vi "Meas_Sweep.vi"(0 "SPU":refnum<k24>, 1 "Flag_215":bool, 2 "MPM":refnum<k24>[](array[refnum]), 3 "Data_struct":refnum<k24>[](array[refnum]), 4 "TSL":refnum<k24>, 5 "错误输入（无错误）":errorcluster, 7 "ILSTS":refnum<k24>, 8 "Flag_213":bool, 11 "Meas_monitor_struct":refnum<k24>[](array[refnum]), 12 "Meas_rang":i32[](array[numeric])) -> (19 "错误输出":errorcluster)   [LabVIEW 2017]
uses:
  D:/test/ILSTS/LV_IL_Sample/DLL/InstrumentDLL.dll
  DLL/InstrumentDLL.dll
  D:/test/ILSTS/LV_IL_Sample/DLL/STSProcess.dll
  DLL/STSProcess.dll
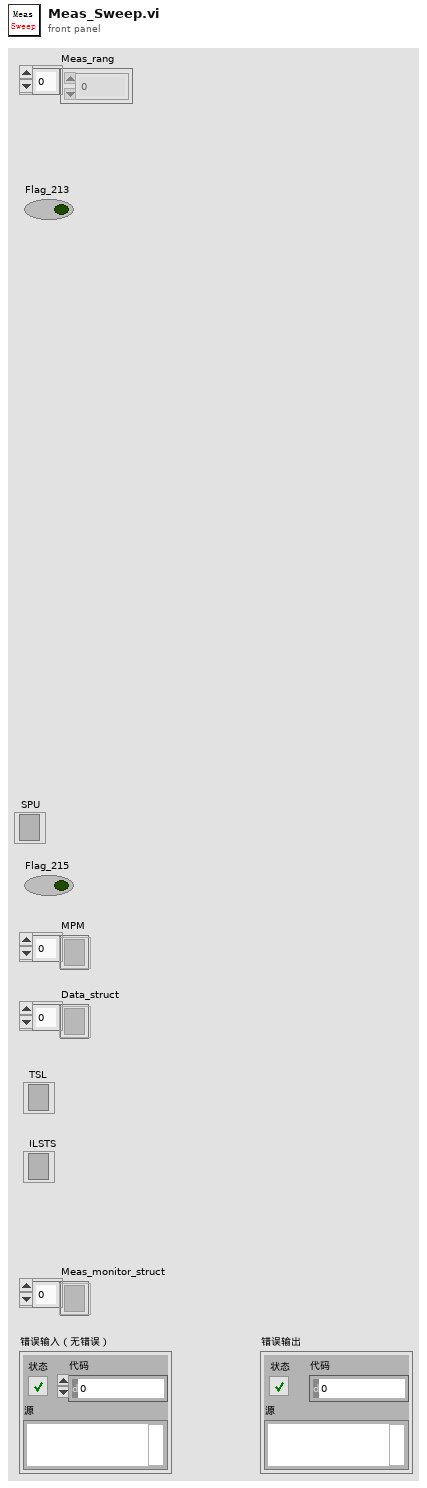
[diagram p1: front panel]
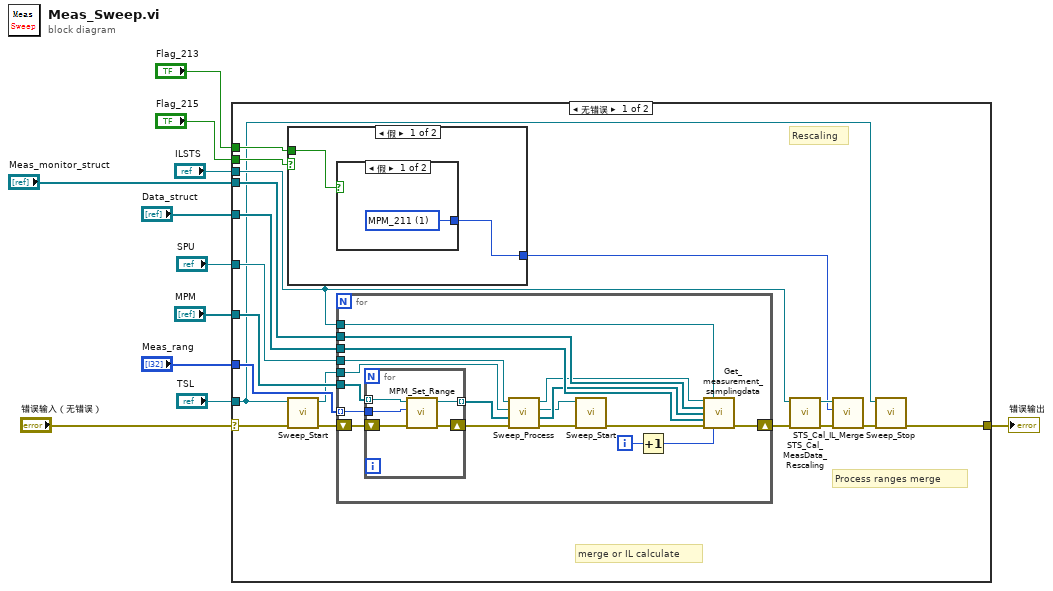
[diagram p0: block diagram]
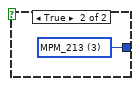
[diagram p2: hidden frame]
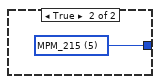
[diagram p3: hidden frame]
diagram:
  n1 = case shown="无错误" "错误输入（无错误）" {
    selector: "错误输入（无错误）" -> [w19 w58]
    tunnel: [w29 w58] -> w11
    tunnel: "Flag_213" -> [w28 _]
    tunnel: "Flag_215" -> [w27 _]
    tunnel: "MPM" -> [w26 _]
    tunnel: "Data_struct" -> [w25 _]
    tunnel: "Meas_monitor_struct" -> [w24 _]
    tunnel: "SPU" -> [w23 _]
    tunnel: "ILSTS" -> [w22 _]
    tunnel: "Meas_rang" -> [w21 _]
    tunnel: "TSL" -> [w20 _]
    frame No Error {
      # "Rescaling"
      # "Process ranges merge"
      # "merge or IL calculate"
      n2 = case shown="假" w27 {
        tunnel: [w31 w34] -> w13
        tunnel: w28 -> [w30 _]
        frame False {
          n3 = case shown="假" w30 {
            tunnel: [w32 w33] -> w31
            frame False {
              w32 = 1 items=["MPM_10"=0, "MPM_211"=1, "MPM_212"=2, "MPM_213"=3, "MPM_215"=5] ("type")
            }
            frame True {
              w33 = 3 items=["MPM_10"=0, "MPM_211"=1, "MPM_212"=2, "MPM_213"=3, "MPM_215"=5] ("type")
            }
          }
        }
        frame True {
          w34 = 5 items=["MPM_10"=0, "MPM_211"=1, "MPM_212"=2, "MPM_213"=3, "MPM_215"=5] ("type")
        }
      }
      n4 = call "Sweep_Start.vi"("error in (no error)"=w19, ".NET Reference in"=w20) -> ("error out"=w18:errorcluster, "Reference out"=w17:refnum<k24>)  [unwired: 8 in]
      n5 = for {
        tunnel: w21 -> [w51] mode=indexing
        tunnel: w26 -> [w43]
        tunnel: w17 -> [w48]
        tunnel: w23 -> [w44]
        tunnel: w22 -> [w47]
        tunnel: w24 -> [w46]
        tunnel: w25 -> [w45]
        shift-right: [w42] -> w12
        shift-left: w18 -> [w52]
        i -> [w41]
        n6 = for {
          tunnel: w43 -> [w57] mode=indexing
          tunnel: w51 -> [w54]
          shift-right: [w55] -> w50
          shift-left: w52 -> [w56]
          tunnel: [w53] -> w40 mode=indexing
          n7 = call "MPM_Set_Range.vi"("error in (no error)"=w56, "Range All"=w54, ".NET Reference in"=w57) -> ("error out"=w55:errorcluster, "Reference out"=w53:refnum<k24>)  [unwired: 7 in]
        }
        n8 = call "Sweep_Process.vi"("错误输入（无错误）"=w50, "MPM"=w40, "TSL"=w48, "SPU"=w44) -> ("error out"=w49:errorcluster, "MPM out"=w39:refnum<k24>[], "TSL out"=w38:refnum<k24>, "SPU out"=w37:refnum<k24>)  [unwired: 4 in]
        n9 = call "Sweep_Start.vi"("error in (no error)"=w49, ".NET Reference in"=w38) -> ("error out"=w36:errorcluster)  [unwired: 8 in, 1 out]
        n10 = Increment(x=w41) -> (x+1=w35:i32)
        n11 = call "Get_measurement_samplingdata.vi"("SPU"=w37, "STSProcess.ILSTS"=w47, "Meas_monitor_struct"=w46, "MPM"=w39, "Data_struct"=w45, "错误输入（无错误）"=w36, "SweepCount"=w35) -> ("error out"=w42:errorcluster)  [unwired: 8 in]
      }
      n12 = call "STS_Cal_MeasData_Rescaling.vi"("错误输入（无错误）"=w12, ".NET引用句柄输入"=w22) -> ("error out"=w14:errorcluster, "引用输出"=w15:refnum<k24>)  [unwired: 8 in]
      n13 = call "STS_Cal_IL_Merge.vi"("错误输入（无错误）"=w14, "type"=w13, ".NET引用句柄输入"=w15) -> ("error out"=w16:errorcluster)  [unwired: 7 in, 1 out]
      n14 = call "Sweep_Stop.vi"("error in (no error)"=w16, ".NET Reference in"=w20) -> ("error out"=w29:errorcluster)  [unwired: 8 in, 1 out]
    }
    frame Error {
    }
  }
  "错误输出" <- w11
